vi "Strip String Quotes.vi"(7 "Skip Type Check? (F)":bool, 11 "JSON":string) -> (3 "Quotes Stripped":string)   [LabVIEW 2020, in "JSON.lvlib"]
uses:
  JSON.lvlib
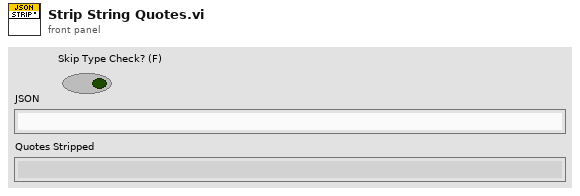
[diagram p1: front panel]
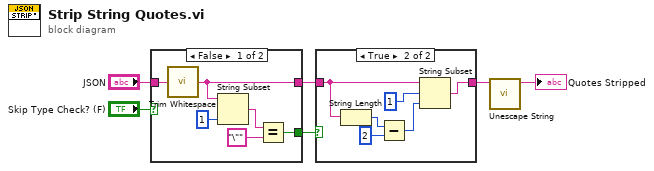
[diagram p0: block diagram]
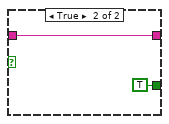
[diagram p2: hidden frame]
diagram:
  n1 = case shown="False" "Skip Type Check? (F)" {
    tunnel: "JSON" -> [w12 w14]
    tunnel: [w10 w14] -> w5
    tunnel: [w7 TRUE] -> w4
    frame False {
      n2 = call <vilib>:"Trim Whitespace.vi"("string"=w12) -> ("trimmed string"=w10:string)  [unwired: 1 in]
      n3 = String Subset(string=w10, length (rest)=1 ("length (rest)")) -> (substring=w9:string)  [unwired: 1 in]
      n4 = Equal?(x=w9, y="\"") -> (x = y?=w7:bool)
    }
    frame True {
    }
  }
  n5 = case shown="True" w4 {
    tunnel: w5 -> [w15 w19]
    tunnel: [w15 w16] -> w2
    frame False {
    }
    frame True {
      n6 = String Length(string=w19) -> (length=w21:i32)
      n7 = Subtract(x=w21, y=2) -> (x-y=w18:i32)
      n8 = String Subset(string=w19, offset (0)=1, length (rest)=w18) -> (substring=w16:string)
    }
  }
  n9 = call "Unescape String.vi"("Escaped String"=w2) -> ("String"=→"Quotes Stripped":string)  [unwired: 10 in]
